vi "Find Support Path.vi"(8 "error in (no error)":errorcluster, 10 "Application Root Folder Name":string, 11 "System Actor in":refnum<class "System Actor.lvclass">) -> (0 "error out":errorcluster, 3 "System Actor out":refnum<class "System Actor.lvclass">)   [LabVIEW 2024, in "System Actor.lvclass"]
uses:
  System Actor.lvclass
  System Actor.lvclass/System Actor.ctl
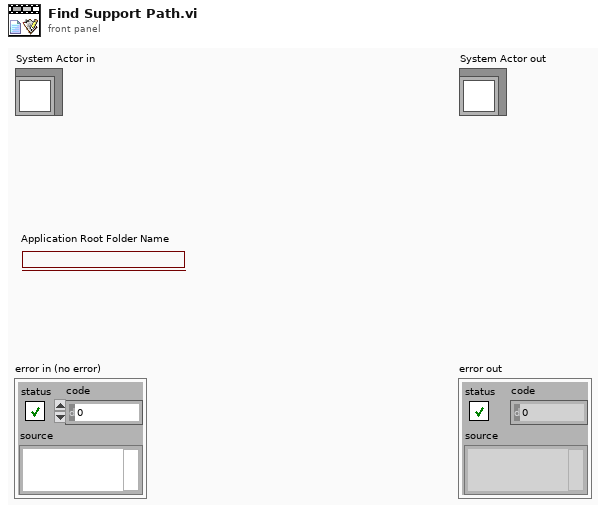
[diagram p1: front panel]
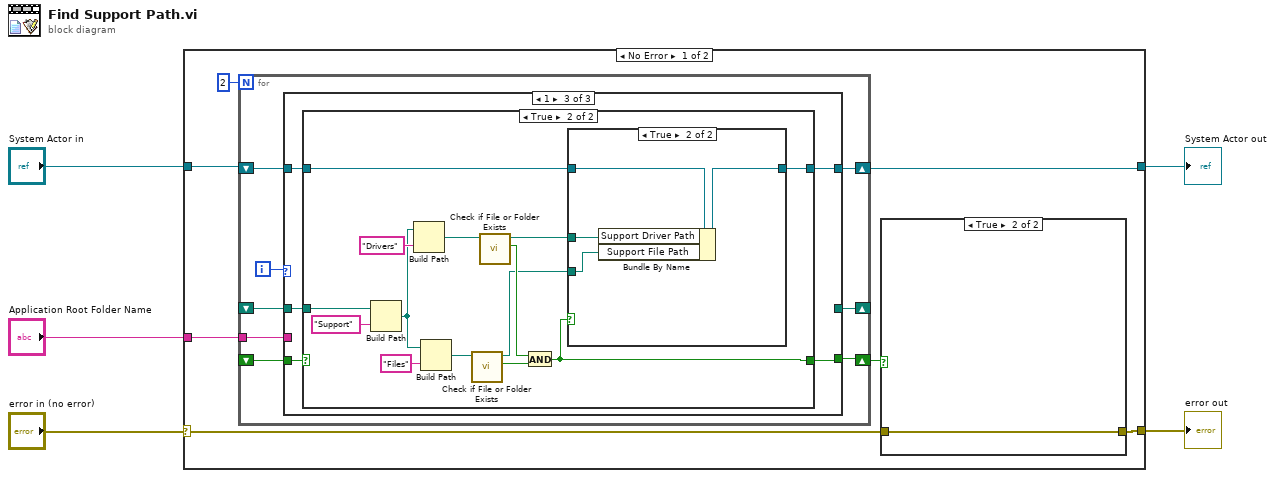
[diagram p0: block diagram]
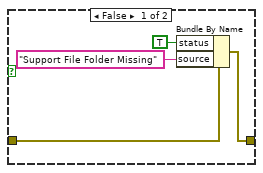
[diagram p2: hidden frame]
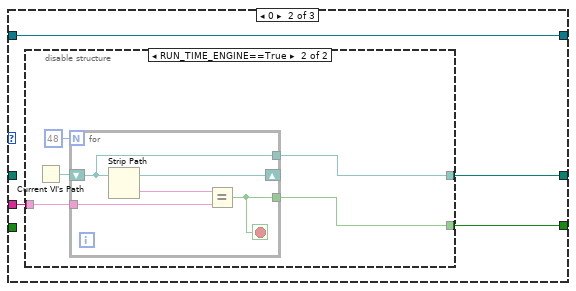
[diagram p4: hidden frame]
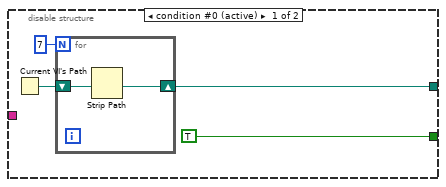
[diagram p5: hidden frame]
diagram:
  n1 = case shown="No Error" "error in (no error)" {
    selector: "error in (no error)" -> [w9 w74]
    tunnel: [w7 w74] -> w4
    tunnel: [w10 w73] -> w2
    tunnel: "System Actor in" -> [w11 w73]
    tunnel: "Application Root Folder Name" -> [w6 _]
    frame No Error {
      n2 = for {
        N: 2 -> [_]
        shift-right: [w24] -> w10
        shift-left: w11 -> [w23]
        shift-right: [w25] -> w8
        shift-left: _ -> [w21]
        shift-right: [w20] -> _
        shift-left: _ -> [w19]
        tunnel: w6 -> [w18]
        i -> [w22]
        n3 = case shown="1" w22 {
          tunnel: [_ w30 w50] -> w25
          tunnel: [w26 w29 w47] -> w24
          tunnel: w23 -> [w26 w29 w48]
          tunnel: w21 -> [_ _ w51]
          tunnel: [_ w28 _] -> w20
          tunnel: w19 -> [_ _ w49]
          tunnel: w18 -> [_ w27 _]
          frame -1, Default {
          }
          frame 0 {
            n4 = disable-structure shown="RUN_TIME_ENGINE==True" {
              disable-tunnel: [w32 w38] -> w28
              disable-tunnel: [TRUE w39] -> w30
              disable-tunnel: w27 -> [_ w41]
              frame condition #0 (active) {
                n5 = Current VI's Path() -> (path=w34:path)
                n6 = for {
                  N: 7 -> [_]
                  shift-right: [w35] -> w32
                  shift-left: w34 -> [w36]
                  n7 = Strip Path(path=w36) -> (stripped path=w35:path)  [unwired: 1 out]
                }
              }
              frame condition #1 {
                n8 = Current VI's Path() -> (path=w37:path)
                n9 = for {
                  N: 48 -> [_]
                  shift-right: [w46] -> _
                  shift-left: w37 -> [w42]
                  tunnel: w41 -> [w44]
                  tunnel: [w43] -> w39
                  tunnel: [w42] -> w38
                  stop <- w43 stop-if-true
                  n10 = Strip Path(path=w42) -> (stripped path=w46:path, name=w45:string)
                  n11 = Equal?(x=w45, y=w44) -> (x = y?=w43:bool)
                }
              }
            }
          }
          frame 1 {
            n12 = case shown="True" w51 {
              selector: w51 -> [w53 _]
              tunnel: [w53 w61] -> w50
              tunnel: w49 -> [_ w66]
              tunnel: w48 -> [w52 w62]
              tunnel: [w52 w59] -> w47
              frame False {
              }
              frame True {
                n13 = Build Path(base path=w66, name or relative path="Support") -> (appended path=w55:path)
                n14 = Build Path(base path=w55, name or relative path="Drivers") -> (appended path=w58:path)
                n15 = Build Path(base path=w55, name or relative path="Files") -> (appended path=w56:path)
                n16 = call <vilib>:"Check if File or Folder Exists.vi"("path"=w56) -> ("file or folder exists?"=w64:bool, "dup path"=w60:path)  [unwired: 8 in, 1 out]
                n17 = call <vilib>:"Check if File or Folder Exists.vi"("path"=w58) -> ("file or folder exists?"=w65:bool, "dup path"=w63:path)  [unwired: 8 in, 1 out]
                n18 = And(x=w65, y=w64) -> (x .and. y?=w61:bool)
                n19 = case shown="True" w61 {
                  tunnel: w63 -> [_ w71]
                  tunnel: w62 -> [w68 w72]
                  tunnel: w60 -> [_ w70]
                  tunnel: [w68 w69] -> w59
                  frame False {
                  }
                  frame True {
                    n20 = Bundle By Name(cluster=w72, "Support Driver Path"=w71, "Support File Path"=w70) -> (w69:refnum<class "System Actor.lvclass">)
                  }
                }
              }
            }
          }
        }
      }
      n21 = case shown="True" w8 {
        tunnel: w9 -> [w16 w17]
        tunnel: [w15 w17] -> w7
        frame False {
          n22 = Bundle By Name(cluster=w16, "status"=TRUE, "source"="Support File Folder Missing") -> (w15:errorcluster)
        }
        frame True {
        }
      }
    }
    frame Error {
    }
  }
  "error out" <- w4
  "System Actor out" <- w2
